vi "integal_caribat_squence.vi"(0 "inner_b_ir":dbl, 1 "inner_f_ir":dbl, 2 "target_ir_l":dbl, 3 "target_ir_r":dbl, 4 "precision":dbl) -> ()   [LabVIEW 2017]
uses:
  Untitled Project 6/GlobalVar.vi
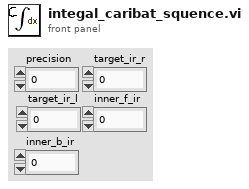
[diagram p1: front panel]
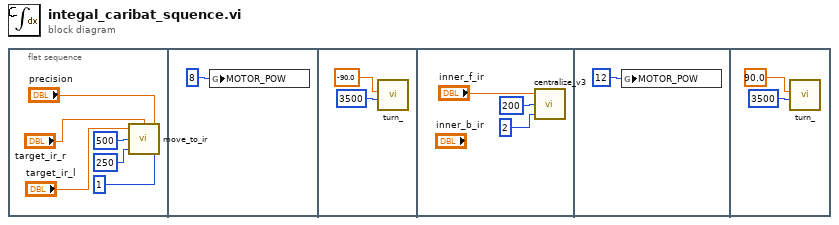
[diagram p0: block diagram]
diagram:
  n1 = flat-sequence {
    frame #0 {
      n2 = call "move_to_ir.vi"("step"=1, "precision"="precision", "target_ir_r"="target_ir_r", "samples"=250, "delay_after"=u32 500, "target_ir_l"="target_ir_l") -> ()
    }
    frame #1 {
      n3 = global write "GlobalVar.vi" "MOTOR_POW"(i8 8 ("MOTOR_POW")) -> ()
    }
    frame #2 {
      n4 = call "turn_.vi"("delay"=u32 3500, "Carzeta"=-90.0) -> ()  [unwired: 10 in]
    }
    frame #3 {
      n5 = call "centralize_v3.vi"("step(mm)"=2, "samples"=200, "inner_f_ir"="inner_f_ir") -> ()
    }
    frame #4 {
      n6 = global write "GlobalVar.vi" "MOTOR_POW"(i8 12 ("MOTOR_POW")) -> ()
    }
    frame #5 {
      n7 = call "turn_.vi"("delay"=u32 3500, "Carzeta"=90.0) -> ()  [unwired: 10 in]
    }
  }
